vi "Write Layout.vi"(10 "Layout":refnum<class "Layout.lvclass">, 11 "Log Sinks in":refnum<class "Log Sinks.lvclass">) -> (3 "Log Sinks out":refnum<class "Log Sinks.lvclass">)   [LabVIEW 2019, in "TSC Event Logger.lvlib" / "Log Sinks.lvclass"]
doc: "Set the layout type for the sink.\n\n<b>Code Developed By:</b>\nTechnology Service Corporation\nBloomington, IN 47403\nwww.tsc.com/atcs\n\nDeveloper:\nDaniel Coons"
uses:
  Log Sinks.lvclass
  Layouts/Layout.lvclass
  Log Sinks.lvclass/Log Sinks.ctl
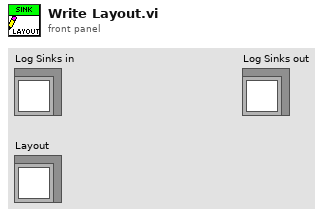
[diagram p1: front panel]
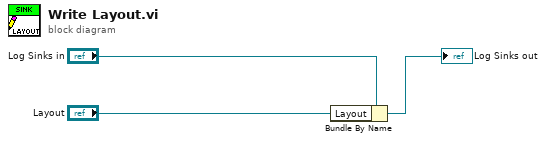
[diagram p0: block diagram]
diagram:
  n1 = Bundle By Name(cluster="Log Sinks in", "Layout"="Layout") -> (→"Log Sinks out":refnum<class "Log Sinks.lvclass">)
